vi "PPG_ABC.get default letter.vi"(0 "i ref in":refnum<vi>, 5 "error in (no error)":errorcluster) -> (14 "i ref out":refnum<vi>, 15 "letter":string, 16 "patternGroup":i32, 19 "error out":errorcluster)   [LabVIEW 2014, in "PPG_ABC.lvlib"]
doc: "Gets name of the default letter that will be used when executing the next SetTime command.A letter has the format XN, where X denotes a letter between A and Z and N denotes the \"memory index\" (not the number of the time table) starting at 1."
uses:
  PPG_ABC.lvlib
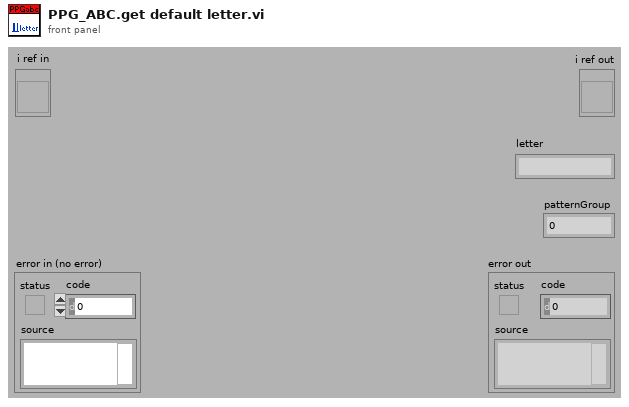
[diagram p1: front panel]
types:
  T1 = typedef "PPG_ABC.lvlib/PPG_ABC.i attribute.ctl" = cluster{"patternGroups":T2[], "defaultLetter":string, "defaultPatternGroup":i32, "PGRunning":T3, "PGRunningID":i32, "pgStarting":T4}
  T2 = typedef "PPG_ABC.lvlib/PPG_ABC.PG_dataType.ctl" = cluster{"PGDevice":string, "rawPatternData":cluster{"triggerCondition":i32, "timeTable":dbl[], "channelTable":string[]}[]}
  T3 = typedef "PPG_ABC.lvlib/PPG_ABC.PG_Running.ctl" = i32
  T4 = typedef "Semaphore RefNum" = refnum<k1>
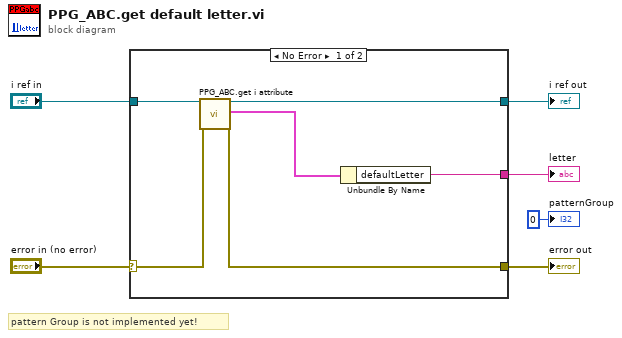
[diagram p0: block diagram]
diagram:
  # "pattern Group is not implemented yet!"
  n1 = case shown="No Error" "error in (no error)" {
    selector: "error in (no error)" -> [w10 w14]
    tunnel: [w9 w14] -> w5
    tunnel: "i ref in" -> [w12 w13]
    tunnel: [w11 w13] -> w3
    tunnel: [w7 _] -> w2
    frame No Error {
      n2 = call "PPG_ABC.get i attribute.vi"("i ref in"=w12, "error in (no error)"=w10) -> ("i ref out"=w11:refnum<vi>, "i attribute"=w8:T1, "error out"=w9:errorcluster)  [unwired: 15 in]
      n3 = Unbundle By Name(w8) -> ("defaultLetter"=w7:string)
    }
    frame Error {
    }
  }
  "error out" <- w5
  "i ref out" <- w3
  "letter" <- w2
  "patternGroup" <- 0 ("patternGroup")
